vi "Run Service.vi"() -> ()   [LabVIEW 2020, in "Line Regulation.lvlib"]
uses:
  Line Regulation.lvlib
  RPC Service/ServiceManagementService/ServiceManagementService.lvclass
  C:/Program Files/National Instruments/LabVIEW 2020/vi.lib/gRPC/LabVIEW gRPC Servicer/ServiceBase/ServiceBase.lvclass
  RPC Service/MeasurementService/MeasurementService.lvclass
  <vilib>/gRPC/LabVIEW gRPC Servicer/Servicer/Servicer.lvclass/Servicer.ctl
  <vilib>/gRPC/LabVIEW gRPC Servicer/Servicer/Servicer.lvclass
  <vilib>/TAF/Discovery Client/Discovery_client.lvlib
panel:
  out "Listening Port":i32
  in  "Stop":bool
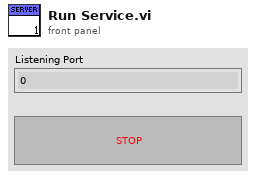
[diagram p1: front panel]
types:
  T1 = typedef "gprc-lvsupport-release.lvlib/grpcId.ctl" = u64
  T2 = typedef "Discovery_client.lvlib/NIMeasurementServices_RegisterServiceResponse.ctl" = cluster{"registration_id":string}
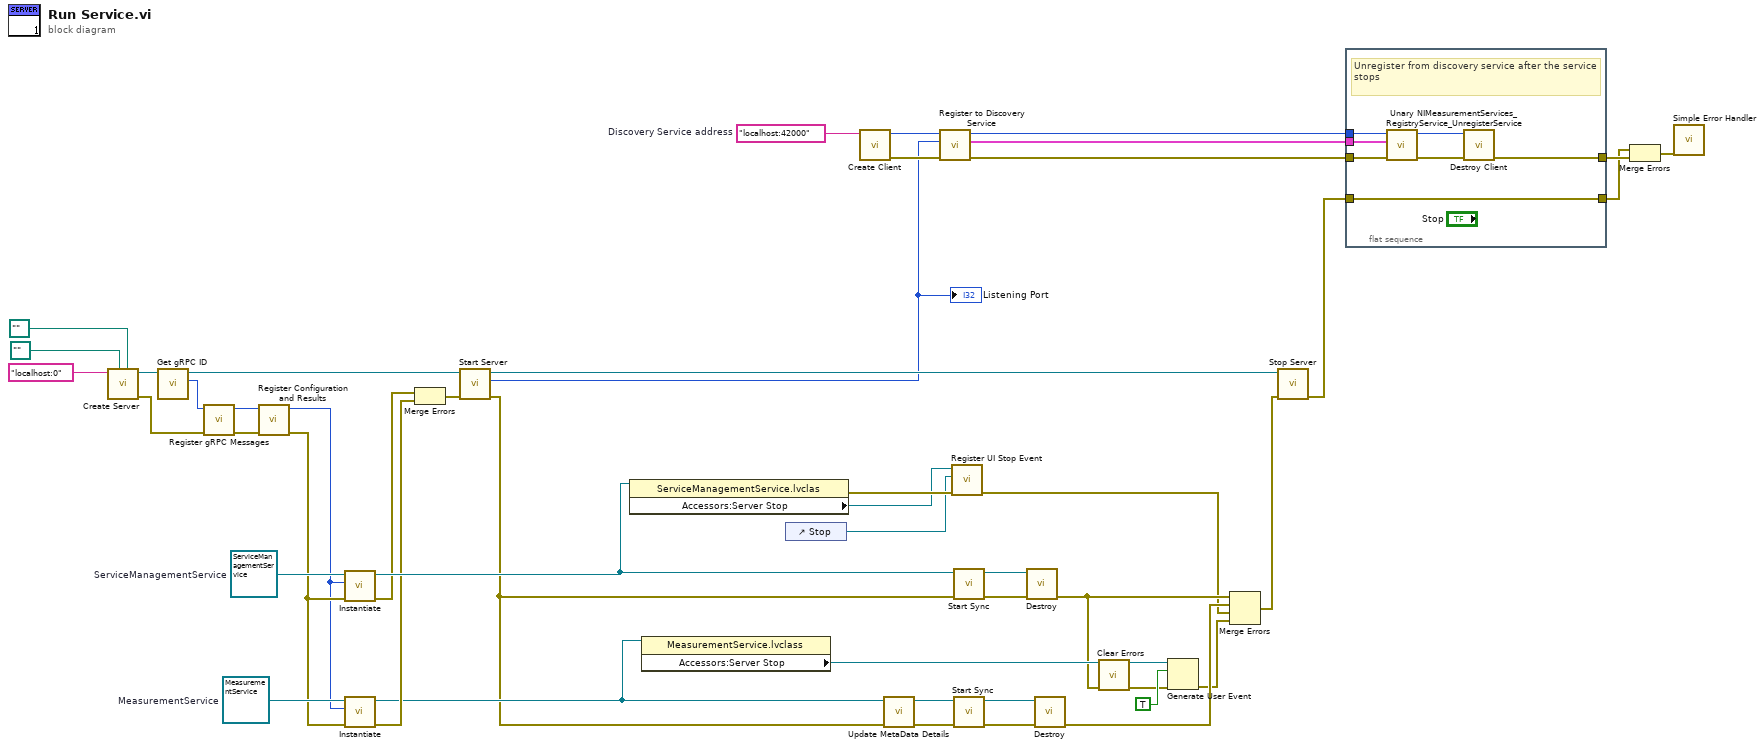
[diagram p0: block diagram]
diagram:
  w29 = "localhost:42000"  # Discovery Service address
  w35 = refnum<class "MeasurementService.lvclass"> refnum  # MeasurementService
  w38 = refnum<class "ServiceManagementService.lvclass"> refnum  # ServiceManagementService
  n1 = call <vilib>:"Create Server.vi"("Server Key File (.key)"=path "", "Server Certificate File (.crt)"=path "", "Server Address"="localhost:0") -> ("error out"=w42:errorcluster, "gRPC Server out"=w44:refnum<class "Servicer.lvclass">)  [unwired: 7 in]
  n2 = call <vilib>:"Get gRPC ID.vi"("OOP Server in"=w44) -> ("gRPC ID"=w43:T1, "OOP Server out"=w34:refnum<class "Servicer.lvclass">)  [unwired: 9 in]
  n3 = call "Register gRPC Messages.vi"("error in (no error)"=w42, "gRPC ID"=w43) -> ("error out"=w11:errorcluster, "gRPC ID Out"=w12:T1)  [unwired: 8 in]
  n4 = call "Register Configuration and Results.vi"("error in (no error)"=w11, "gRPC ID"=w12) -> ("error out"=w10:errorcluster, "gRPC ID Out"=w4:T1)  [unwired: 8 in]
  n5 = call-dynamic "Instantiate.vi"("error in (no error)"=w10, "gRPCid"=w4, "iService"=w38) -> ("error out"=w26:errorcluster, "iService"=w41:refnum<class "ServiceManagementService.lvclass">)  [unwired: 7 in]
  n6 = call-dynamic "Instantiate.vi"("error in (no error)"=w10, "gRPCid"=w4, "iService"=w35) -> ("error out"=w28:errorcluster, "iService"=w9:refnum<class "MeasurementService.lvclass">)  [unwired: 7 in]
  n7 = Merge Errors(w26, w28) -> (w27:errorcluster)
  n8 = call <vilib>:"Start Server.vi"("error in (no error)"=w27, "gRPC Server in"=w34) -> ("error out"=w7:errorcluster, "Listening Port"=w5:i32, "gRPC Server out"=w48:refnum<class "Servicer.lvclass">)  [unwired: 7 in]
  "Listening Port" <- w5
  n9 = property class="ServiceManagementService.lvclas"(reference=w41) -> (error out=w19:errorcluster, "Accessors:Server Stop"=w18:refnum<user-event>)  [unwired: 1 in, 1 out]
  n10 = property class="MeasurementService.lvclass"(reference=w9) -> ("Accessors:Server Stop"=w33:refnum<user-event>)  [unwired: 1 in, 2 out]
  n11 = control-ref of="Stop"() -> (w17:refnum<vi>)
  n12 = call <vilib>:"Create Client.vi"("address"=w29) -> ("error out"=w23:errorcluster, "gRPC ID Out"=w24:T1)  [unwired: 9 in]
  n13 = call "Update MetaData Details.vi"("error in"=w7, "MeasurementService.lvclass"=w9) -> ("error out"=w6:errorcluster, "MeasurementService.lvclass"=w8:refnum<class "MeasurementService.lvclass">)  [unwired: 8 in]
  n14 = call "Register to Discovery Service.vi"("error in"=w23, "PortNumber"=w5, "gRPC ID"=w24) -> ("error out"=w21:errorcluster, "Response Data"=w20:T2, "gRPC ID out"=w22:T1)  [unwired: 6 in]
  n15 = call "Register UI Stop Event.vi"("error in"=w19, "Stop Button [ref]"=w17, "Server Stop"=w18) -> ("error out"=w1:errorcluster)  [unwired: 8 in]
  n16 = call-dynamic "Start Sync.vi"("error in (no error)"=w7, "gRPC Server in"=w41) -> ("error out"=w39:errorcluster, "gRPC Server out"=w40:refnum<class "ServiceManagementService.lvclass">)  [unwired: 8 in]
  n17 = call-dynamic "Start Sync.vi"("error in (no error)"=w6, "gRPC Server in"=w8) -> ("error out"=w37:errorcluster, "gRPC Server out"=w36:refnum<class "MeasurementService.lvclass">)  [unwired: 8 in]
  n18 = call-dynamic "Destroy.vi"("error in (no error)"=w39, "SignalGeneratorService in"=w40) -> ("error out"=w31:errorcluster)  [unwired: 8 in, 1 out]
  n19 = call-dynamic "Destroy.vi"("error in (no error)"=w37, "SignalGeneratorService in"=w36) -> ("error out"=w3:errorcluster)  [unwired: 8 in, 1 out]
  n20 = call <vilib>:"Clear Errors.vi"("error in (no error)"=w31) -> ("error out"=w30:errorcluster)  [unwired: 5 in, 1 out]
  n21 = Generate User Event(user event=w33, event data cluster=TRUE ("event data"), error in=w30) -> (error out=w2:errorcluster)  [unwired: 1 in, 1 out]
  n22 = Merge Errors(w31, w3, w1, w2) -> (w25:errorcluster)
  n23 = call <vilib>:"Stop Server.vi"("error in (no error)"=w25, "gRPC Server in"=w48) -> ("error out"=w13:errorcluster)  [unwired: 9 in]
  n24 = flat-sequence {
    tunnel: w22 -> [w55]
    tunnel: w21 -> [w54]
    tunnel: w20 -> [w53]
    tunnel: [w50] -> w16
    tunnel: [w49] -> w14
    tunnel: w13 -> [w49]
    frame #0 {
      # "Unregister from discovery service after the service stops"
      n25 = call <vilib>:"Unary NIMeasurementServices_RegistryService_UnregisterService.vi"("error in"=w54, "Request Data"=w53, "gRPC ID"=w55) -> ("error out"=w51:errorcluster, "gRPC ID out"=w52:T1)  [unwired: 6 in, 1 out]
      n26 = call <vilib>:"Destroy Client.vi"("error in"=w51, "gRPC ID"=w52) -> ("error out"=w50:errorcluster)  [unwired: 9 in]
    }
  }
  n27 = Merge Errors(w14, w16) -> (w15:errorcluster)
  n28 = call <vilib>:"Simple Error Handler.vi"("error in (no error)"=w15) -> ()  [unwired: 4 in, 5 out]
